vi "Set Package License.vi"(8 "error in (no error)":errorcluster, 10 "License":string, 11 "PackageInfo in":refnum<class "PackageInfo.lvclass">) -> (0 "error out":errorcluster, 3 "PackageInfo out":refnum<class "PackageInfo.lvclass">)   [LabVIEW 2020, in "GPack.lvlib" / "PackageInfo.lvclass"]
uses:
  PackageInfo.lvclass
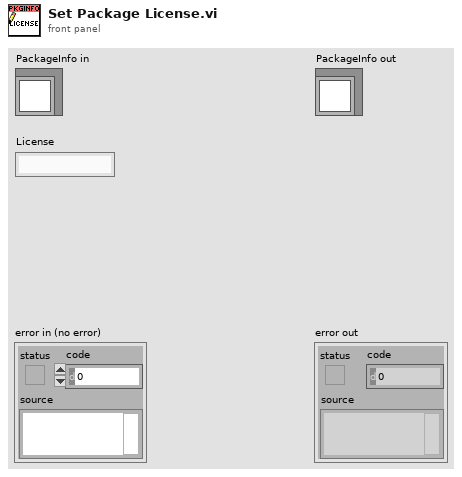
[diagram p1: front panel]
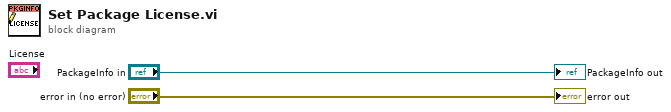
[diagram p0: block diagram]
diagram:
  "error out" <- "error in (no error)"
  "PackageInfo out" <- "PackageInfo in"
